vi "GetTemp.vi"() -> (0 "result":dbl format="%.4f")   [LabVIEW 2014]
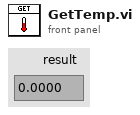
[diagram p1: front panel]
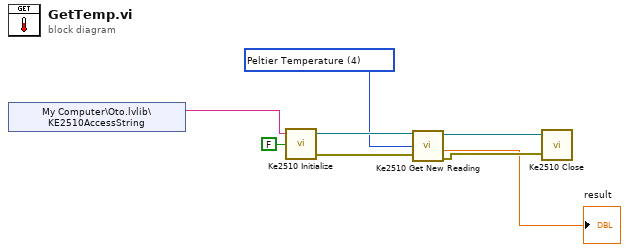
[diagram p0: block diagram]
diagram:
  w4 = 4 items=["Peltier DC Current", "Peltier Power", "Peltier DC Resistance", "Peltier AC Resistance", "Peltier Temperature", "Peltier DC Voltage", "Sensor Temperature"] ("function")
  n1 = shared-variable "My Computer\\Oto.lvlib\\KE2510AccessString"() -> (w7:string)  [unwired: 1 in, 1 out]
  n2 = call <instrlib>:"Ke2510 Initialize.vi"("reset device"=FALSE, "resource name"=w7) -> ("error out"=w5:errorcluster, "instrument handle"=w6:refnum<visa-resource-name>)  [unwired: 1 in, 1 out]
  n3 = call <instrlib>:"Ke2510 Get New Reading.vi"("instrument handle"=w6, "function"=w4, "error in (no error)"=w5) -> ("instrument handle out"=w3:refnum<visa-resource-name>, "result"=→"result":dbl, "error out"=w2:errorcluster)  [unwired: 1 out]
  n4 = call <instrlib>:"Ke2510 Close.vi"("instrument handle"=w3, "error in (no error)"=w2) -> ()  [unwired: 1 in, 2 out]
